vi "rs3 init all2.vi"(8 "error in":errorcluster, 10 "Select Device":i32, 11 "Select Sensor":i32) -> (0 "error out":errorcluster, 1 "Adv. enable?":i32, 2 "init results":T3, 3 "init error":string, 4 "All Devices":T2(array[cluster]), 5 "Sensor Array":T1(array[cluster]), 7 "Found RealSense":bool)   [LabVIEW 2017, in "libRealSense3.lvlib"]
doc: "Initialized the RealSense device. \nSelect the specific DEVICE and its specific SENSOR. \n\n\nINPUT:\nSelect Device The INDEX to the specific DEVICE handle\nSelect Sensor The INDEX to the specific SENSOR that is part of the selected DEVICE.\n \nOUTPUT:\ninit result Contains all the information about the selected device and its sensor. You will need to use the Dev Out HANDLE to communicate with the device. \n \nselected sensor array Contains the arrays of SENSORS attached to a specific DEVICE.\nall devices Contains array of all device that are attached to the PC."
uses:
  libRealSense3.lvlib
panel:
  # "RS3 Init All"
  # "(C) Intel Corp. 2017,  AGJ"
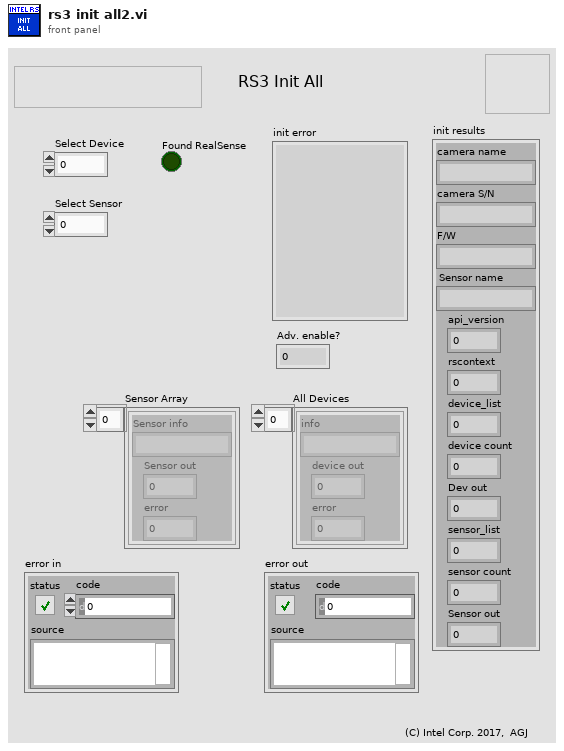
[diagram p1: front panel]
types:
  T1 = cluster{"Sensor info":string, "Sensor out":u64, "error":u64}[]
  T2 = cluster{"info":string, "device out":u64, "error":u64}[]
  T3 = cluster{"camera name":string, "camera S/N":string, "F/W":string, "Sensor name":string, "api_version":i32, "rscontext":u64, "device_list":u64, "device count":i32, "Dev out":u64, "sensor_list":u64, "sensor count":i32, "Sensor out":u64}
  T4 = cluster{"info":string, "device out":u64, "error":u64}
  T5 = cluster{"info":string, "info":string, "info":string, "Sensor info":string, "api_version":i32, "rscontext":u64, "device_list":u64, "device count":i32, "device out":u64, "sensor_list":u64, "sensor count":i32, "Sensor out":u64}
  T6 = cluster{"Sensor info":string, "Sensor out":u64, "error":u64}
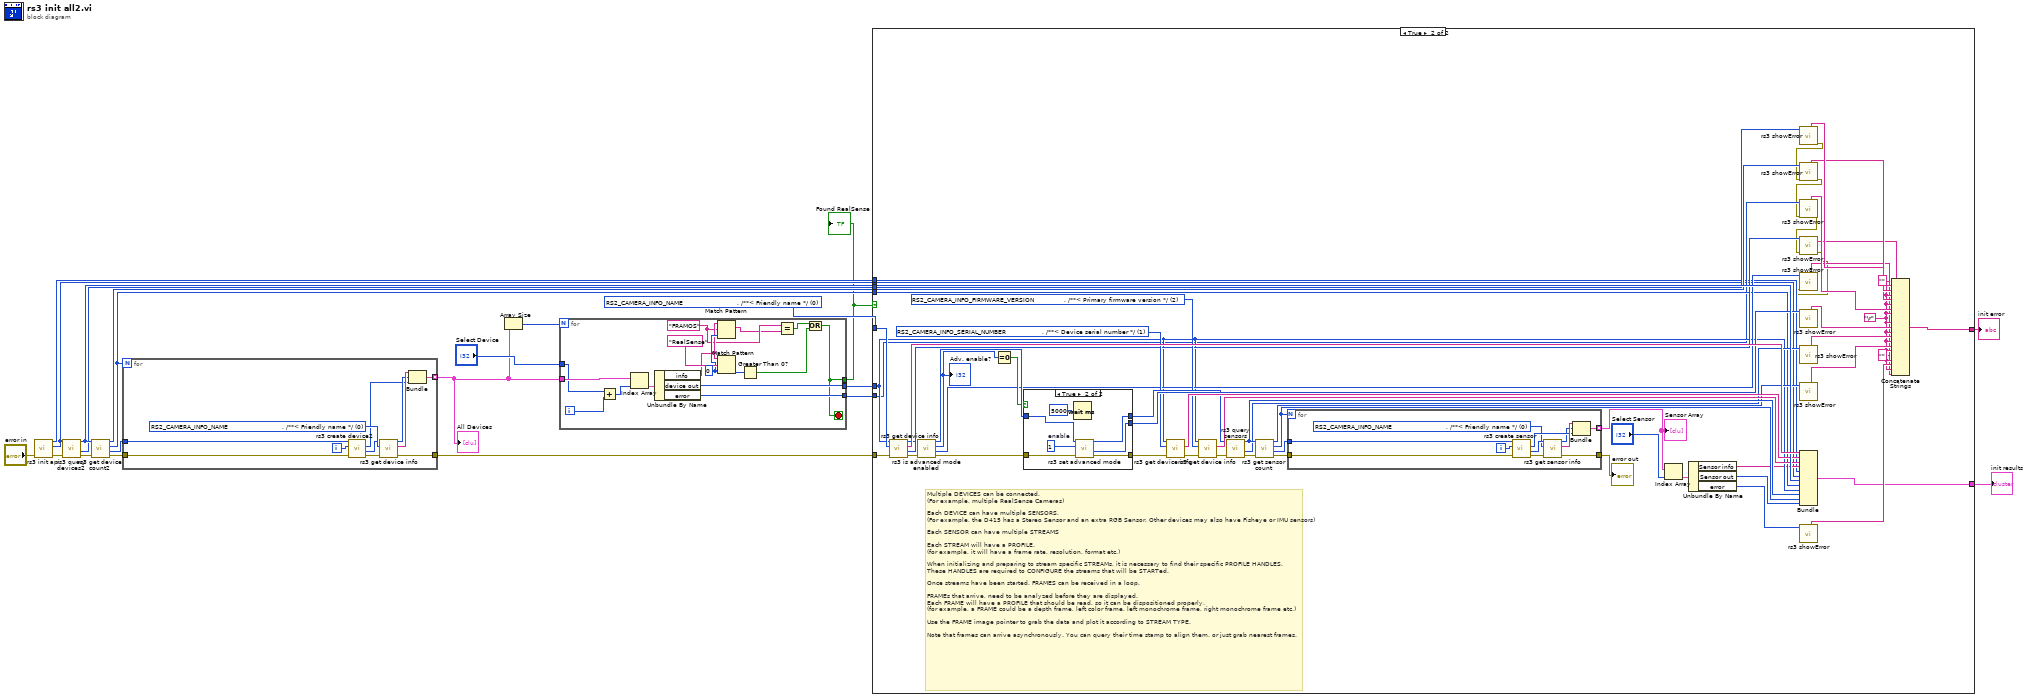
[diagram p0: block diagram]
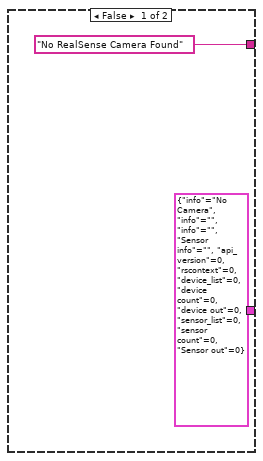
[diagram p2: hidden frame]
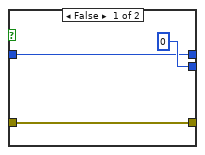
[diagram p3: hidden frame]
diagram:
  w20 = u16 0 items=["    RS2_CAMERA_INFO_NAME                           , /**< Friendly name */", "    RS2_CAMERA_INFO_SERIAL_NUMBER                  , /**< Device serial number */", "    RS2_CAMERA_INFO_FIRMWARE_VERSION               , /**< Primary firmware version */", "    RS2_CAMERA_INFO_PHYSICAL_PORT                       , /**< Unique identifier of the port the device is connected to (platform specific) */", "    RS2_CAMERA_INFO_DEBUG_OP_CODE                  , /**< If device supports firmware logging, this is the command to send to get logs from firmware */", "    RS2_CAMERA_INFO_ADVANCED_MODE                  , /**< True iff the device is in advanced mode */", "    RS2_CAMERA_INFO_PRODUCT_ID                     , /**< Product ID as reported in the USB descriptor */", "    RS2_CAMERA_INFO_CAMERA_LOCKED                  , /**< True iff EEPROM is locked */", "    RS2_CAMERA_INFO_COUNT                            /**< Number of enumeration values. Not a valid input: intended to be used in for-loops. */"] ("RS Camera info")
  n1 = call "rs3 init api.vi"("error in (no error)"="error in") -> ("error out"=w9:errorcluster, "rscontext"=w7:u64, "api_version"=w6:i32)  [unwired: 7 in, 1 out]
  n2 = call "rs3 query devices2.vi"("error in (no error)"=w9, "rscontext"=w7) -> ("error out"=w18:errorcluster, "error"=w17:u64, "device_list"=w21:u64)  [unwired: 7 in]
  n3 = call "rs3 get device count2.vi"("error in"=w18, "device_list"=w21) -> ("error out"=w12:errorcluster, "device_list_out"=w15:u64, "device count"=w16:i32, "error"=w19:u64)  [unwired: 6 in]
  n4 = for {
    N: w16 -> [_]
    tunnel: w15 -> [w32]
    tunnel: [w26] -> w1 mode=indexing
    tunnel: w12 -> [w25]
    tunnel: [w24] -> w11
    i -> [w31]
    w29 = u16 0 items=["    RS2_CAMERA_INFO_NAME                           , /**< Friendly name */", "    RS2_CAMERA_INFO_SERIAL_NUMBER                  , /**< Device serial number */", "    RS2_CAMERA_INFO_FIRMWARE_VERSION               , /**< Primary firmware version */", "    RS2_CAMERA_INFO_PHYSICAL_PORT                       , /**< Unique identifier of the port the device is connected to (platform specific) */", "    RS2_CAMERA_INFO_DEBUG_OP_CODE                  , /**< If device supports firmware logging, this is the command to send to get logs from firmware */", "    RS2_CAMERA_INFO_ADVANCED_MODE                  , /**< True iff the device is in advanced mode */", "    RS2_CAMERA_INFO_PRODUCT_ID                     , /**< Product ID as reported in the USB descriptor */", "    RS2_CAMERA_INFO_CAMERA_LOCKED                  , /**< True iff EEPROM is locked */", "    RS2_CAMERA_INFO_COUNT                            /**< Number of enumeration values. Not a valid input: intended to be used in for-loops. */"] ("RS Camera info")
    n5 = call "rs3 create device2.vi"("error in (no error)"=w25, "Device index"=w31, "device list in"=w32) -> ("error out"=w30:errorcluster, "Dev out"=w23:u64, "error"=w22:u64)  [unwired: 5 in, 1 out]
    n6 = call "rs3 get device info.vi"("error in (no error)"=w30, "RS Camera info"=w29, "device in"=w23) -> ("error out"=w24:errorcluster, "info"=w28:string, "device out"=w27:u64)  [unwired: 5 in, 1 out]
    n7 = Bundle("info"=w28, "device out"=w27, "error"=w22) -> (w26:T4)  [unwired: 1 in]
  }
  "All Devices" <- w1
  n8 = Array Size(array=w1) -> (size(s)=w2:i32)
  n9 = for {
    N: w2 -> [_]
    tunnel: w1 -> [w48]
    tunnel: "Select Device" -> [w41]
    tunnel: [w46] -> w13
    tunnel: [w45] -> w10
    tunnel: [w37] -> w5
    i -> [w42]
    stop <- w37 stop-if-true
    w34 = "FRAMOS"
    w39 = 0 ("offset (0)")
    n10 = Add(x=w41, y=w42) -> (x+y=w43:i32)
    n11 = Index Array(array=w48, index=w43) -> (element=w47:T4)
    n12 = Unbundle By Name(w47) -> ("info"=w36:string, "device out"=w46:u64, "error"=w45:u64)
    n13 = Match Pattern(string=w36, regular expression=w34, offset (0)=w39) -> (match substring=w33:string)  [unwired: 3 out]
    n14 = Match Pattern(string=w36, regular expression="RealSense" ("string"), offset (0)=w39) -> (offset past match=w40:i32)  [unwired: 3 out]
    n15 = Greater Than 0?(x=w40) -> (x > 0?=w38:bool)
    n16 = Equal?(x=w34, y=w33) -> (x = y?=w35:bool)
    n17 = Or(x=w35, y=w38) -> (x .or. y?=w37:bool)
  }
  "Found RealSense" <- w5
  n18 = case shown="True" w5 {
    tunnel: w21 -> [_ w108]
    tunnel: w20 -> [_ w95]
    tunnel: w19 -> [_ w93]
    tunnel: w17 -> [_ w92]
    tunnel: w16 -> [_ w74]
    tunnel: w13 -> [_ w73]
    tunnel: w11 -> [_ w72]
    tunnel: w10 -> [_ w71]
    tunnel: w7 -> [_ w60]
    tunnel: w6 -> [_ w59]
    tunnel: ["No RealSense Camera Found" w58] -> w4
    tunnel: [T5 {"info"="No Camera", "info"="", "info"="", "Sensor info"="", "api_version"=0, "rscontext"=0, "device_list"=0, "device count"=0, "device out"=0, "sensor_list"=0, "sensor count"=0, "Sensor out"=0} w57] -> w3
    frame False {
    }
    frame True {
      w76 = "\r"
      w102 = u16 2 items=["    RS2_CAMERA_INFO_NAME                           , /**< Friendly name */", "    RS2_CAMERA_INFO_SERIAL_NUMBER                  , /**< Device serial number */", "    RS2_CAMERA_INFO_FIRMWARE_VERSION               , /**< Primary firmware version */", "    RS2_CAMERA_INFO_PHYSICAL_PORT                       , /**< Unique identifier of the port the device is connected to (platform specific) */", "    RS2_CAMERA_INFO_DEBUG_OP_CODE                  , /**< If device supports firmware logging, this is the command to send to get logs from firmware */", "    RS2_CAMERA_INFO_ADVANCED_MODE                  , /**< True iff the device is in advanced mode */", "    RS2_CAMERA_INFO_PRODUCT_ID                     , /**< Product ID as reported in the USB descriptor */", "    RS2_CAMERA_INFO_CAMERA_LOCKED                  , /**< True iff EEPROM is locked */", "    RS2_CAMERA_INFO_COUNT                            /**< Number of enumeration values. Not a valid input: intended to be used in for-loops. */"] ("RS Camera info")
      w101 = u16 1 items=["    RS2_CAMERA_INFO_NAME                           , /**< Friendly name */", "    RS2_CAMERA_INFO_SERIAL_NUMBER                  , /**< Device serial number */", "    RS2_CAMERA_INFO_FIRMWARE_VERSION               , /**< Primary firmware version */", "    RS2_CAMERA_INFO_PHYSICAL_PORT                       , /**< Unique identifier of the port the device is connected to (platform specific) */", "    RS2_CAMERA_INFO_DEBUG_OP_CODE                  , /**< If device supports firmware logging, this is the command to send to get logs from firmware */", "    RS2_CAMERA_INFO_ADVANCED_MODE                  , /**< True iff the device is in advanced mode */", "    RS2_CAMERA_INFO_PRODUCT_ID                     , /**< Product ID as reported in the USB descriptor */", "    RS2_CAMERA_INFO_CAMERA_LOCKED                  , /**< True iff EEPROM is locked */", "    RS2_CAMERA_INFO_COUNT                            /**< Number of enumeration values. Not a valid input: intended to be used in for-loops. */"] ("RS Camera info")
      # "Multiple DEVICES can be connected. \n(For example, multiple RealSense Cameras)\n\nEach DEVICE can have multiple SENSORS. \n(For example, the D415 has a Stereo Sensor and an extra RGB Sensor. Other devices may also have Fisheye or IMU sensors) \n\nEach SENSOR can have multiple STREAMS\n\nEach STREAM will have a PROFILE. \n(for example, it will have a frame rate, resolution, format etc.)\n\nWhen initializing and preparing to stream specific STREAMs, it is necessary to find their specific PROFILE HANDLES.\nThese HANDLES are required to CONFIGURE the streams that will be STARTed. \n\nOnce streams have been started, FRAMES can be received in a loop. \n \nFRAMEs that arrive, need to be analyzed before they are displayed. \nEach FRAME will have a PROFILE that should be read, so it can be dispositioned properly.\n(for example, a FRAME could be a depth frame, left color frame, left monochrome frame, right monochrome frame etc.)\n\nUse the FRAME image pointer to grab the data and plot it according to STREAM TYPE.\n\nNote that frames can arrive asynchronously. You can query their time stamp to align them, or just grab nearest frames."
      n19 = call "rs3 get device info.vi"("error in (no error)"=w72, "RS Camera info"=w95, "device in"=w73) -> ("error out"=w83:errorcluster, "error"=w94:u64, "info"=w109:string, "device out"=w81:u64)  [unwired: 5 in]
      n20 = call "rs3 is advanced mode enabled.vi"("error in (no error)"=w83, "device in"=w81) -> ("error out"=w82:errorcluster, "error"=w77:u64, "enable?"=w79:i32, "device out"=w80:u64)  [unwired: 6 in]
      "Adv. enable?" <- w79
      n21 = Equal To 0?(x=w79) -> (x = 0?=w78:bool)
      n22 = case shown="True" w78 {
        tunnel: [u64 0 ("error") w131] -> w105
        tunnel: [w122 w129] -> w104
        tunnel: w80 -> [w122 w128]
        tunnel: [w124 w127] -> w103
        tunnel: w82 -> [w124 w126]
        frame False {
        }
        frame True {
          w130 = 1  # enable
          n23 = Wait (ms)(milliseconds to wait=u32 5000) -> ()  [unwired: 1 out]
          n24 = call "rs3 set advanced mode.vi"("error in (no error)"=w126, "enable"=w130, "device in"=w128) -> ("error out"=w127:errorcluster, "error"=w131:u64, "device out"=w129:u64)  [unwired: 6 in]
        }
      }
      n25 = call "rs3 get device info.vi"("error in (no error)"=w103, "RS Camera info"=w101, "device in"=w73) -> ("error out"=w99:errorcluster, "info"=w106:string)  [unwired: 5 in, 2 out]
      n26 = call "rs3 get device info.vi"("error in (no error)"=w99, "RS Camera info"=w102, "device in"=w73) -> ("error out"=w100:errorcluster, "info"=w107:string)  [unwired: 5 in, 2 out]
      n27 = call "rs3 query sensors.vi"("error in (no error)"=w100, "device in"=w104) -> ("error out"=w97:errorcluster, "error"=w96:u64, "sensor_list"=w110:u64)  [unwired: 7 in]
      n28 = call "rs3 get sensor count.vi"("error in"=w97, "sensor_list"=w110) -> ("error out"=w69:errorcluster, "sensor_list_out"=w68:u64, "sensor count"=w70:i32, "error"=w98:u64)  [unwired: 6 in]
      n29 = for {
        N: w70 -> [_]
        tunnel: w69 -> [w121]
        tunnel: w68 -> [w118]
        tunnel: [w112] -> w67 mode=indexing
        tunnel: [w111] -> w62
        i -> [w119]
        w114 = u16 0 items=["    RS2_CAMERA_INFO_NAME                           , /**< Friendly name */", "    RS2_CAMERA_INFO_SERIAL_NUMBER                  , /**< Device serial number */", "    RS2_CAMERA_INFO_FIRMWARE_VERSION               , /**< Primary firmware version */", "    RS2_CAMERA_INFO_PHYSICAL_PORT                       , /**< Unique identifier of the port the device is connected to (platform specific) */", "    RS2_CAMERA_INFO_DEBUG_OP_CODE                  , /**< If device supports firmware logging, this is the command to send to get logs from firmware */", "    RS2_CAMERA_INFO_ADVANCED_MODE                  , /**< True iff the device is in advanced mode */", "    RS2_CAMERA_INFO_PRODUCT_ID                     , /**< Product ID as reported in the USB descriptor */", "    RS2_CAMERA_INFO_CAMERA_LOCKED                  , /**< True iff EEPROM is locked */", "    RS2_CAMERA_INFO_COUNT                            /**< Number of enumeration values. Not a valid input: intended to be used in for-loops. */"] ("RS Sensor info")
        n30 = call "rs3 create sensor.vi"("error in (no error)"=w121, "Sensor index"=w119, "Sensor list"=w118) -> ("error out"=w120:errorcluster, "Sensor out"=w116:u64, "error"=w115:u64)  [unwired: 5 in, 1 out]
        n31 = call "rs3 get sensor info.vi"("error in (no error)"=w120, "RS Camera info"=w114, "Sensor in"=w116) -> ("error out"=w111:errorcluster, "Sensor info"=w117:string, "Sensor out"=w113:u64)  [unwired: 5 in, 1 out]
        n32 = Bundle("Sensor info"=w117, "Sensor out"=w113, "error"=w115) -> (w112:T6)  [unwired: 1 in]
      }
      "error out" <- w62
      "Sensor Array" <- w67
      n33 = Index Array(array=w67, index="Select Sensor") -> (element=w65:T6)
      n34 = Unbundle By Name(w65) -> ("Sensor info"=w61:string, "Sensor out"=w64:u64, "error"=w63:u64)
      n35 = Bundle("info"=w109, "info"=w106, "info"=w107, "Sensor info"=w61, "api_version"=w59, "rscontext"=w60, "device_list"=w108, "device count"=w74, "device out"=w73, "sensor_list"=w110, "sensor count"=w70, "Sensor out"=w64) -> (w57:T5)  [unwired: 1 in]
      n36 = call "rs3 showError.vi"("error"=w92) -> ("error out"=w56:errorcluster, "Error summary"=w91:string)  [unwired: 6 in, 3 out]
      n37 = call "rs3 showError.vi"("error in (no error)"=w56, "error"=w93) -> ("error out"=w55:errorcluster, "Error summary"=w90:string)  [unwired: 5 in, 3 out]
      n38 = call "rs3 showError.vi"("error in (no error)"=w55, "error"=w71) -> ("error out"=w54:errorcluster, "Error summary"=w89:string)  [unwired: 5 in, 3 out]
      n39 = call "rs3 showError.vi"("error in (no error)"=w54, "error"=w94) -> ("error out"=w53:errorcluster, "Error summary"=w88:string)  [unwired: 5 in, 3 out]
      n40 = call "rs3 showError.vi"("error in (no error)"=w53, "error"=w77) -> ("Error summary"=w75:string)  [unwired: 5 in, 4 out]
      n41 = call "rs3 showError.vi"("error"=w105) -> ("Error summary"=w87:string)  [unwired: 6 in, 4 out]
      n42 = call "rs3 showError.vi"("error"=w96) -> ("Error summary"=w86:string)  [unwired: 6 in, 4 out]
      n43 = call "rs3 showError.vi"("error"=w98) -> ("Error summary"=w85:string)  [unwired: 6 in, 4 out]
      n44 = call "rs3 showError.vi"("error"=w63) -> ("Error summary"=w84:string)  [unwired: 6 in, 4 out]
      n45 = Concatenate Strings("" ("string"), w76, w91, w76, w90, w76, w89, w76, w88, w76, w87, w76, w86, w76, w85, w76, "" ("string"), w76, w84, w76, w75) -> (w58:string)
    }
  }
  "init error" <- w4
  "init results" <- w3
